vi "DHE_fdMgr.vi"(6 "error in (no error)":errorcluster, 8 "Device In":T1 {"readtime" format="%.2f"}, 9 "arg in":string, 10 "action":T2(ring), 11 "cmd in":string) -> (1 "devices":T1[](array[typedef]) {"readtime" format="%.2f"}, 2 "Device":T1 {"readtime" format="%.2f"}, 3 "cmd out":string, 4 "error out":errorcluster)   [LabVIEW 2016]
uses:
  private/vis/DHE_Device.ctl
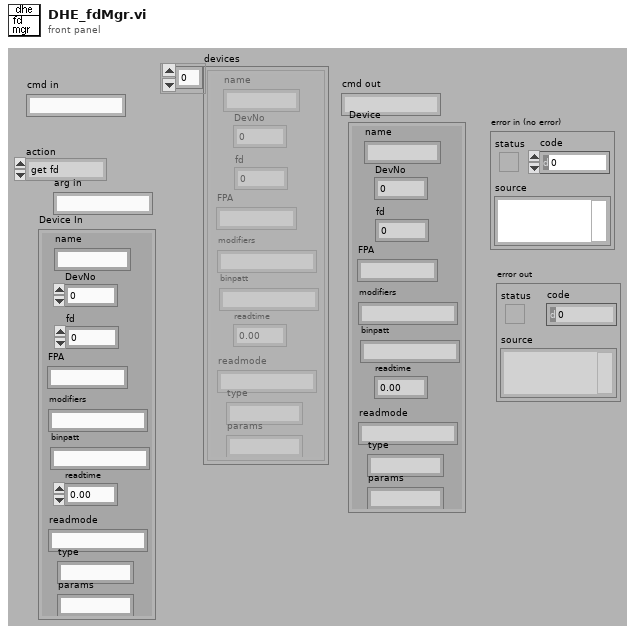
[diagram p1: front panel]
types:
  T1 = typedef "DHE_Device.ctl" = cluster{"DevNo":i32, "fd":i32, "name":string, "FPA":string, "modifiers":string, "binpatt":string, "readtime":dbl, "readmode":string, "type":string, "params":string}
  T2 = enum16{"get fd", "set fd", "add ", "set_readtime", "get all", "clean all", "get by fd"}
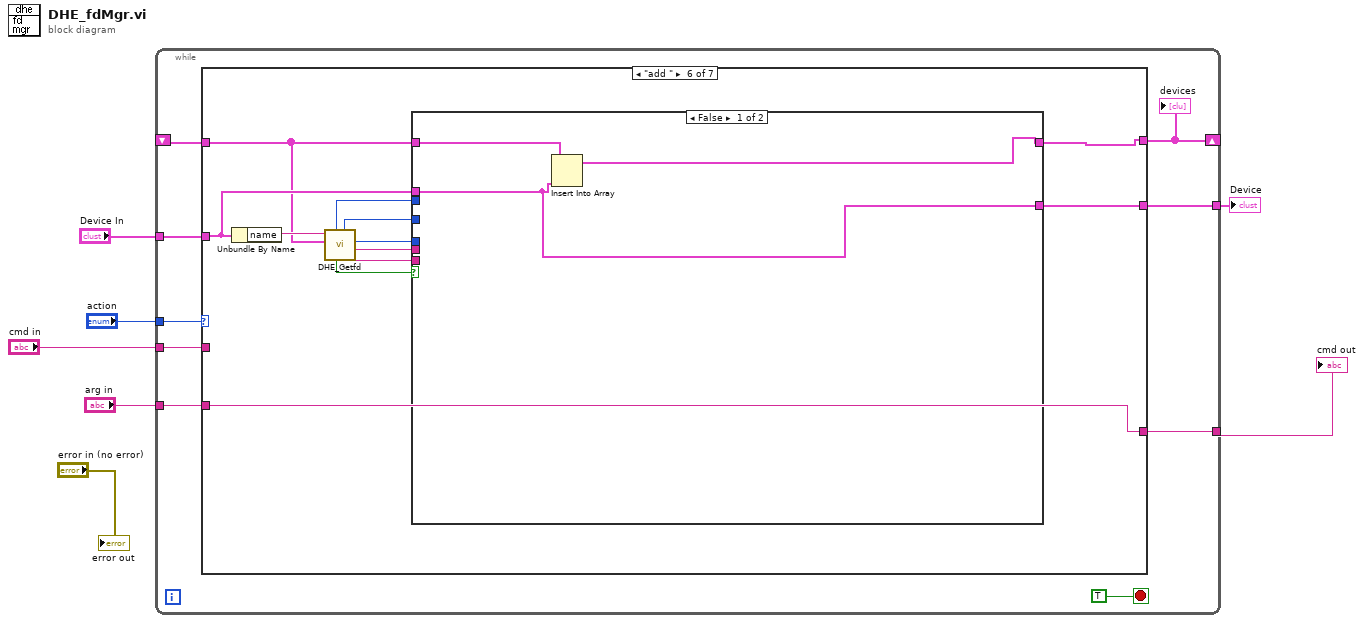
[diagram p0: block diagram]
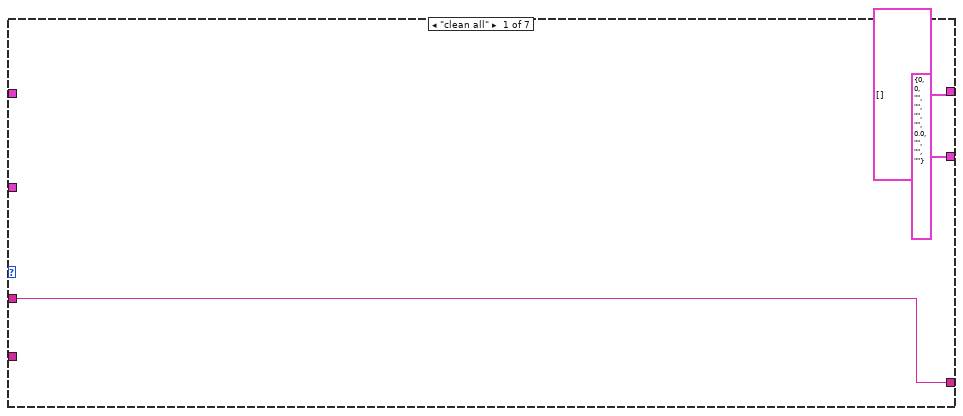
[diagram p2: hidden frame]
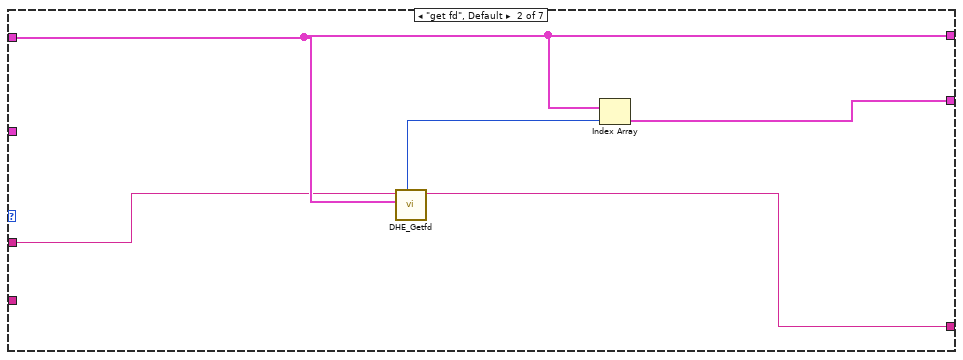
[diagram p3: hidden frame]
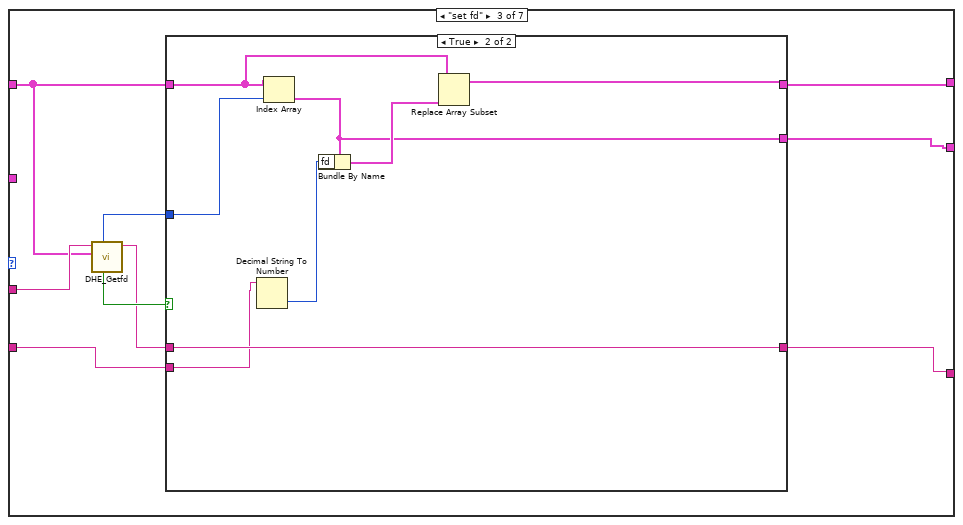
[diagram p4: hidden frame]
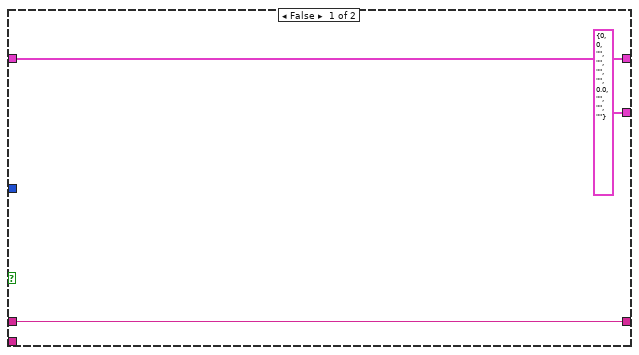
[diagram p5: hidden frame]
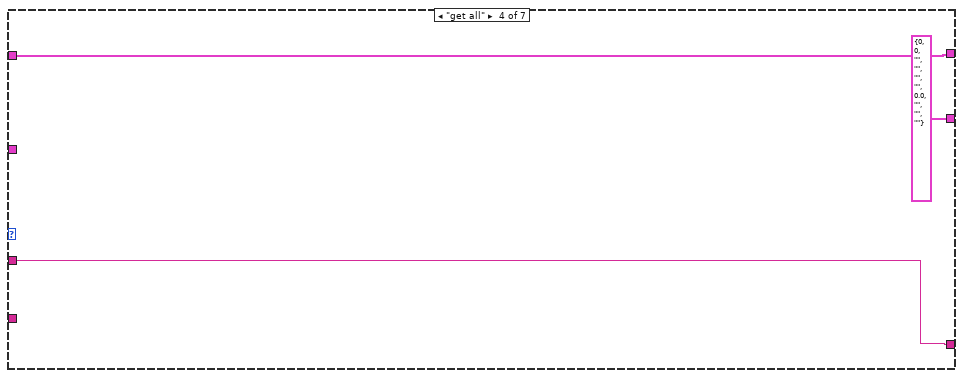
[diagram p6: hidden frame]
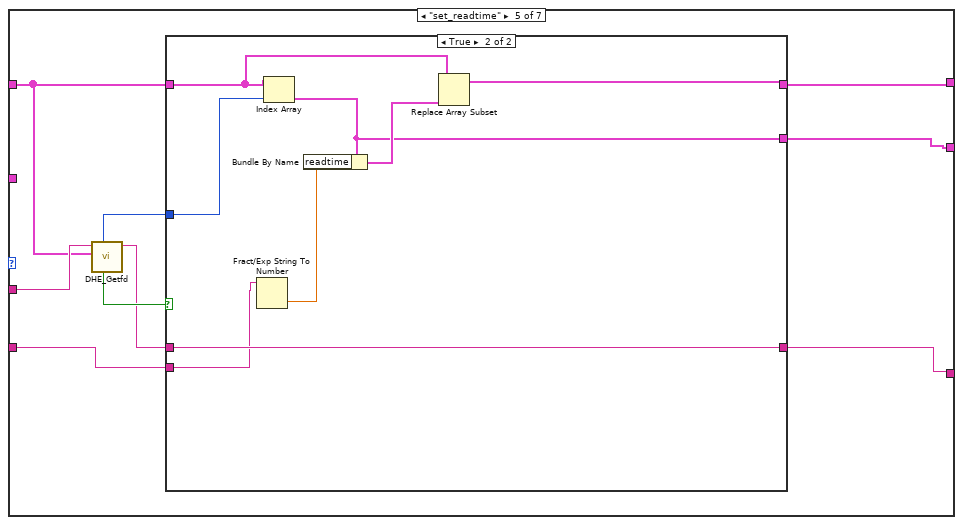
[diagram p7: hidden frame]
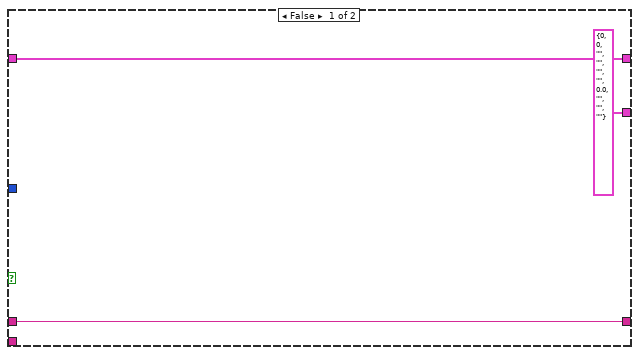
[diagram p8: hidden frame]
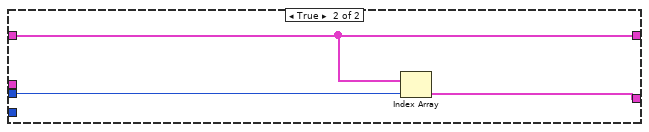
[diagram p9: hidden frame]
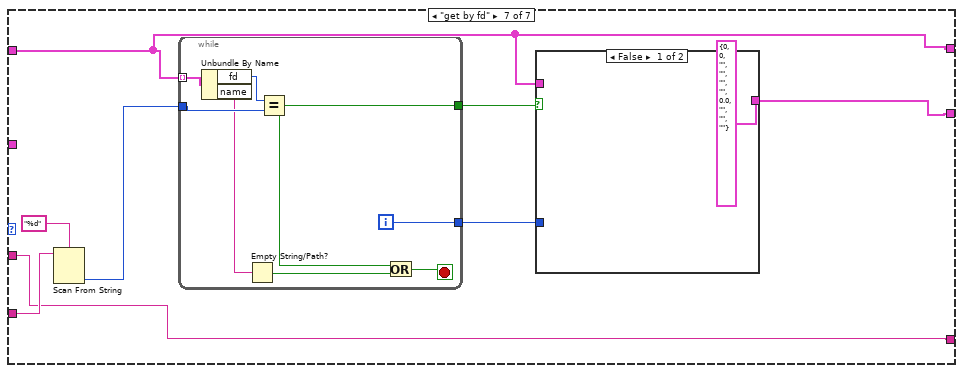
[diagram p10: hidden frame]
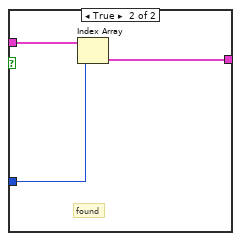
[diagram p11: hidden frame]
diagram:
  n1 = while {
    tunnel: [w16] -> w7
    tunnel: "cmd in" -> [w15]
    tunnel: "action" -> [w13]
    tunnel: "arg in" -> [w12]
    shift-right: [w9] -> _
    shift-left: _ -> [w11]
    tunnel: "Device In" -> [w10]
    tunnel: [w8] -> w2
    stop <- TRUE stop-if-true
    n2 = case shown="\"add \"" w13 {
      tunnel: [w17 w24 w31 w47 w54 w75 w86] -> w16
      tunnel: w15 -> [w17 w20 w33 w47 w56 _ w86]
      tunnel: w11 -> [_ w22 w26 w46 w49 w68 w89]
      tunnel: w12 -> [_ _ w28 _ w51 w75 w87]
      tunnel: [T1[] [] w22 w27 w46 w50 w71 w89] -> w9
      tunnel: w10 -> [_ _ _ _ _ w72 _]
      tunnel: [T1 {"DevNo"=0, "fd"=0, "name"="", "FPA"="", "modifiers"="", "binpatt"="", "readtime"=0.0, "readmode"="", "type"="", "params"=""} ("Device In") w21 w25 T1 {"DevNo"=0, "fd"=0, "name"="", "FPA"="", "modifiers"="", "binpatt"="", "readtime"=0.0, "readmode"="", "type"="", "params"=""} ("Device In") w48 w70 w88] -> w8
      frame "clean all" {
      }
      frame "get fd", Default {
        n3 = call "DHE_Getfd.vi"("DHE_Devices"=w22, "cmd in"=w20) -> ("cmd out"=w24:string, "index"=w23:i32)  [unwired: 8 out]
        n4 = Index Array(array=w22, index=w23) -> (element=w21:T1)
      }
      frame "set fd" {
        n5 = call "DHE_Getfd.vi"("DHE_Devices"=w26, "cmd in"=w33) -> ("cmd out"=w29:string, "found"=w32:bool, "index"=w30:i32)  [unwired: 7 out]
        n6 = case shown="True" w32 {
          tunnel: w26 -> [w36 w43]
          tunnel: [w36 w41] -> w27
          tunnel: w29 -> [w35 w40]
          tunnel: [w35 w40] -> w31
          tunnel: w30 -> [_ w44]
          tunnel: w28 -> [_ w39]
          tunnel: [T1 {"DevNo"=0, "fd"=0, "name"="", "FPA"="", "modifiers"="", "binpatt"="", "readtime"=0.0, "readmode"="", "type"="", "params"=""} ("Device In") w37] -> w25
          frame False {
          }
          frame True {
            n7 = Decimal String To Number(string=w39) -> (number=w38:i32)  [unwired: 3 out]
            n8 = Index Array(array=w43, index=w44) -> (element=w37:T1)
            n9 = Bundle By Name(cluster=w37, "fd"=w38) -> (w42:T1)
            n10 = Replace Array Subset(array=w43, new element=w42) -> (w41:T1[])  [unwired: 1 in]
          }
        }
      }
      frame "get all" {
      }
      frame "set_readtime" {
        n11 = call "DHE_Getfd.vi"("DHE_Devices"=w49, "cmd in"=w56) -> ("cmd out"=w52:string, "found"=w55:bool, "index"=w53:i32)  [unwired: 7 out]
        n12 = case shown="True" w55 {
          tunnel: w49 -> [w59 w66]
          tunnel: [w59 w64] -> w50
          tunnel: w52 -> [w58 w63]
          tunnel: [w58 w63] -> w54
          tunnel: w53 -> [_ w67]
          tunnel: w51 -> [_ w62]
          tunnel: [T1 {"DevNo"=0, "fd"=0, "name"="", "FPA"="", "modifiers"="", "binpatt"="", "readtime"=0.0, "readmode"="", "type"="", "params"=""} ("Device In") w61] -> w48
          frame False {
          }
          frame True {
            n13 = Fract/Exp String To Number(string=w62) -> (number=w60:dbl)  [unwired: 4 out]
            n14 = Index Array(array=w66, index=w67) -> (element=w61:T1)
            n15 = Bundle By Name(cluster=w61, "readtime"=w60) -> (w65:T1)
            n16 = Replace Array Subset(array=w66, new element=w65) -> (w64:T1[])  [unwired: 1 in]
          }
        }
      }
      frame "add " {
        n17 = Unbundle By Name(w72) -> ("name"=w79:string)
        n18 = call "DHE_Getfd.vi"("DHE_Devices"=w68, "cmd in"=w79) -> ("devname"=w77:string, "fd"=w74:i32, "fpa"=w76:string, "devno"=w73:i32, "found"=w78:bool, "index"=w69:i32)  [unwired: 4 out]
        n19 = case shown="False" w78 {
          tunnel: w77 -> [_ _]
          tunnel: w76 -> [_ _]
          tunnel: w74 -> [_ _]
          tunnel: w73 -> [_ _]
          tunnel: w68 -> [w82 w85]
          tunnel: [w81 w85] -> w71
          tunnel: w72 -> [w80 _]
          tunnel: [w80 w83] -> w70
          tunnel: w69 -> [_ w84]
          frame False {
            n20 = Insert Into Array(array=w82, new element=w80) -> (w81:T1[])  [unwired: 1 in]
          }
          frame True {
            n21 = Index Array(array=w85, index=w84) -> (element=w83:T1)
          }
        }
      }
      frame "get by fd" {
        n22 = Scan From String(format string="%d", input string=w87) -> (output 1=w92:i32)  [unwired: 2 in, 4 out]
        n23 = while {
          tunnel: w89 -> [w105] mode=indexing
          tunnel: w92 -> [w103]
          tunnel: [w102] -> w91
          tunnel: [w98] -> w90
          i -> [w98]
          stop <- w99 stop-if-true
          n24 = Unbundle By Name(w105) -> ("fd"=w104:i32, "name"=w101:string)
          n25 = Empty String/Path?(string/path=w101) -> (empty?=w100:bool)
          n26 = Equal?(x=w104, y=w103) -> (x = y?=w102:bool)
          n27 = Or(x=w102, y=w100) -> (x .or. y?=w99:bool)
        }
        n28 = case shown="False" w91 {
          tunnel: w90 -> [_ w96]
          tunnel: w89 -> [_ w97]
          tunnel: [T1 {"DevNo"=0, "fd"=0, "name"="", "FPA"="", "modifiers"="", "binpatt"="", "readtime"=0.0, "readmode"="", "type"="", "params"=""} ("Device In") w95] -> w88
          frame False {
          }
          frame True {
            # "found"
            n29 = Index Array(array=w97, index=w96) -> (element=w95:T1)
          }
        }
      }
    }
    "devices" <- w9
  }
  "cmd out" <- w7
  "Device" <- w2
  "error out" <- "error in (no error)"
